vi "Is Window Being Shown - Get.vi"() -> (0 "Is Window Being Shown?":bool)   [LabVIEW 2023, in "Error Manager.lvlib" / "Error Display Window.lvclass"]
uses:
  Is Window Being Shown (class variable).vi
  New Error Window/_TBD New Error Window.lvclass/_TBD New Error Window.ctl
  Error Display Window.lvclass
  Error Display Window.lvclass/Error Display Window.ctl
panel:
  # "Development\ncontrols/indicators useful for development and testing, but which are not outputs of the VI"
  # "Input\nInputs to the VI"
  # "Output\nOutputs of the VI"
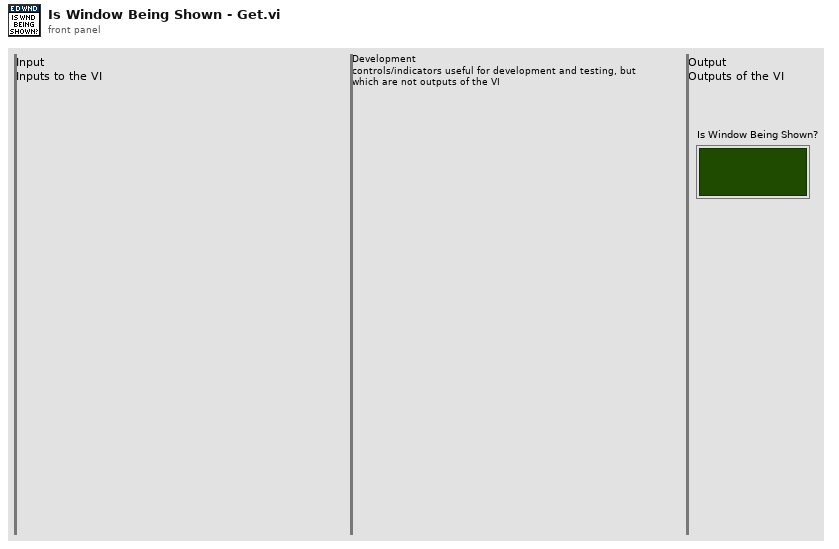
[diagram p1: front panel]
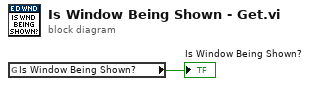
[diagram p0: block diagram]
diagram:
  n1 = global read "Is Window Being Shown (class variable).vi" "Is Window Being Shown?"() -> (→"Is Window Being Shown?":bool)
